vi "WtriteDataTOCheckSNTab.vi"(8 "error in":errorcluster, 11 "SQL":string) -> (0 "error out":errorcluster, 3 "DataOut":string)   [LabVIEW 2013]
uses:
  <vilib>/addons/database/Connection.llb/DB Tools Open Connec (String).vi
  <vilib>/addons/database/Connection.llb/Conn Execute.vi
  <vilib>/addons/database/Recordset.llb/Rec Fetch Recordset Data (R).vi
  <vilib>/addons/database/Recordset.llb/Rec Destroy - Connection.vi
  <vilib>/addons/database/NI_Database_API.lvlib
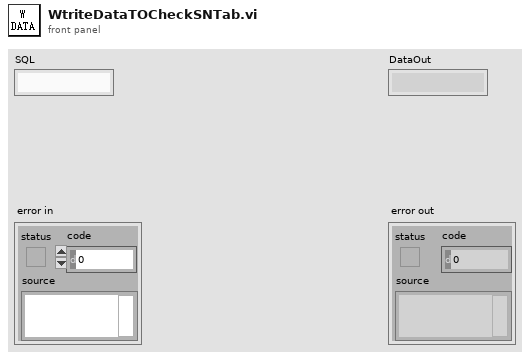
[diagram p1: front panel]
types:
  T1 = typedef "NI_Database_API.lvlib/Conn ObjectReference.ctl" = refnum<k1>
  T2 = typedef "NI_Database_API.lvlib/Rec ObjectReference.ctl" = refnum<k1>
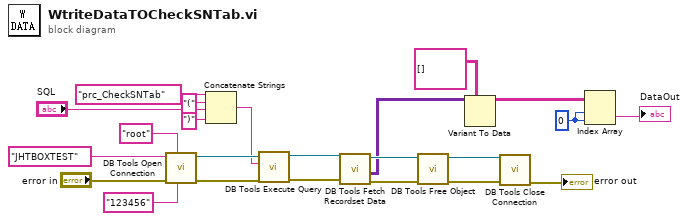
[diagram p0: block diagram]
diagram:
  w2 = 0 ("禁用的索引 (列)")
  n1 = call-poly <vilib>:"DB Tools Open Connection.vi"("password"="123456", "userID"="root", "error in (no error)"="error in", "connection information"="JHTBOXTEST" ("userID")) -> ("error out"=w22:errorcluster, "connection reference"=w23:T1)  [unwired: 4 in]
  n2 = Concatenate Strings("prc_CheckSNTab" ("userID"), "(" ("字符串"), "SQL", ")" ("字符串")) -> (w8:string)
  n3 = call-poly <vilib>:"DB Tools Execute Query.vi"("error in (no error)"=w22, "SQL query"=w8, "connection reference"=w23) -> ("error out"=w21:errorcluster, "recordset reference"=w20:T2)  [unwired: 5 in]
  n4 = call-poly <vilib>:"DB Tools Fetch Recordset Data.vi"("error in (no error)"=w21, "recordset reference"=w20) -> ("error out"=w19:errorcluster, "recordset data"=w5:variant[][], "recordset reference out"=w18:T2)  [unwired: 3 in]
  n5 = call-poly <vilib>:"DB Tools Free Object.vi"("error in (no error)"=w19, "recordset reference"=w18) -> ("error out"=w16:errorcluster, "connection reference"=w17:T1)  [unwired: 8 in]
  n6 = Variant To Data(type=string[][] [] ("数组"), Variant=w5) -> (data=w3:string[][])  [unwired: 1 in, 1 out]
  n7 = call <vilib>:"DB Tools Close Connection.vi"("error in (no error)"=w16, "connection reference"=w17) -> ("error out"=→"error out":errorcluster)  [unwired: 5 in]
  n8 = Index Array(array=w3, index (row)=w2, index (col)=w2) -> (element=→"DataOut":string)
